vi "UpdateCurrent.vi"(8 "error in (no error)":errorcluster) -> (0 "error out":errorcluster)   [LabVIEW 2015]
uses:
  <vilib>/Rock Robotics/WPI/CAN/TalonSRX/WPI_CANTalonSRX_GlobalStatus.ctl
  Shooter Global.vi
panel:
  out "Set Pos":dbl(graph)
  out "Closed Loop Error":dbl(graph)
  out "Encoder Pos":dbl(graph)
  out "Current":dbl(graph)
  out "Talon SRX Status":T1
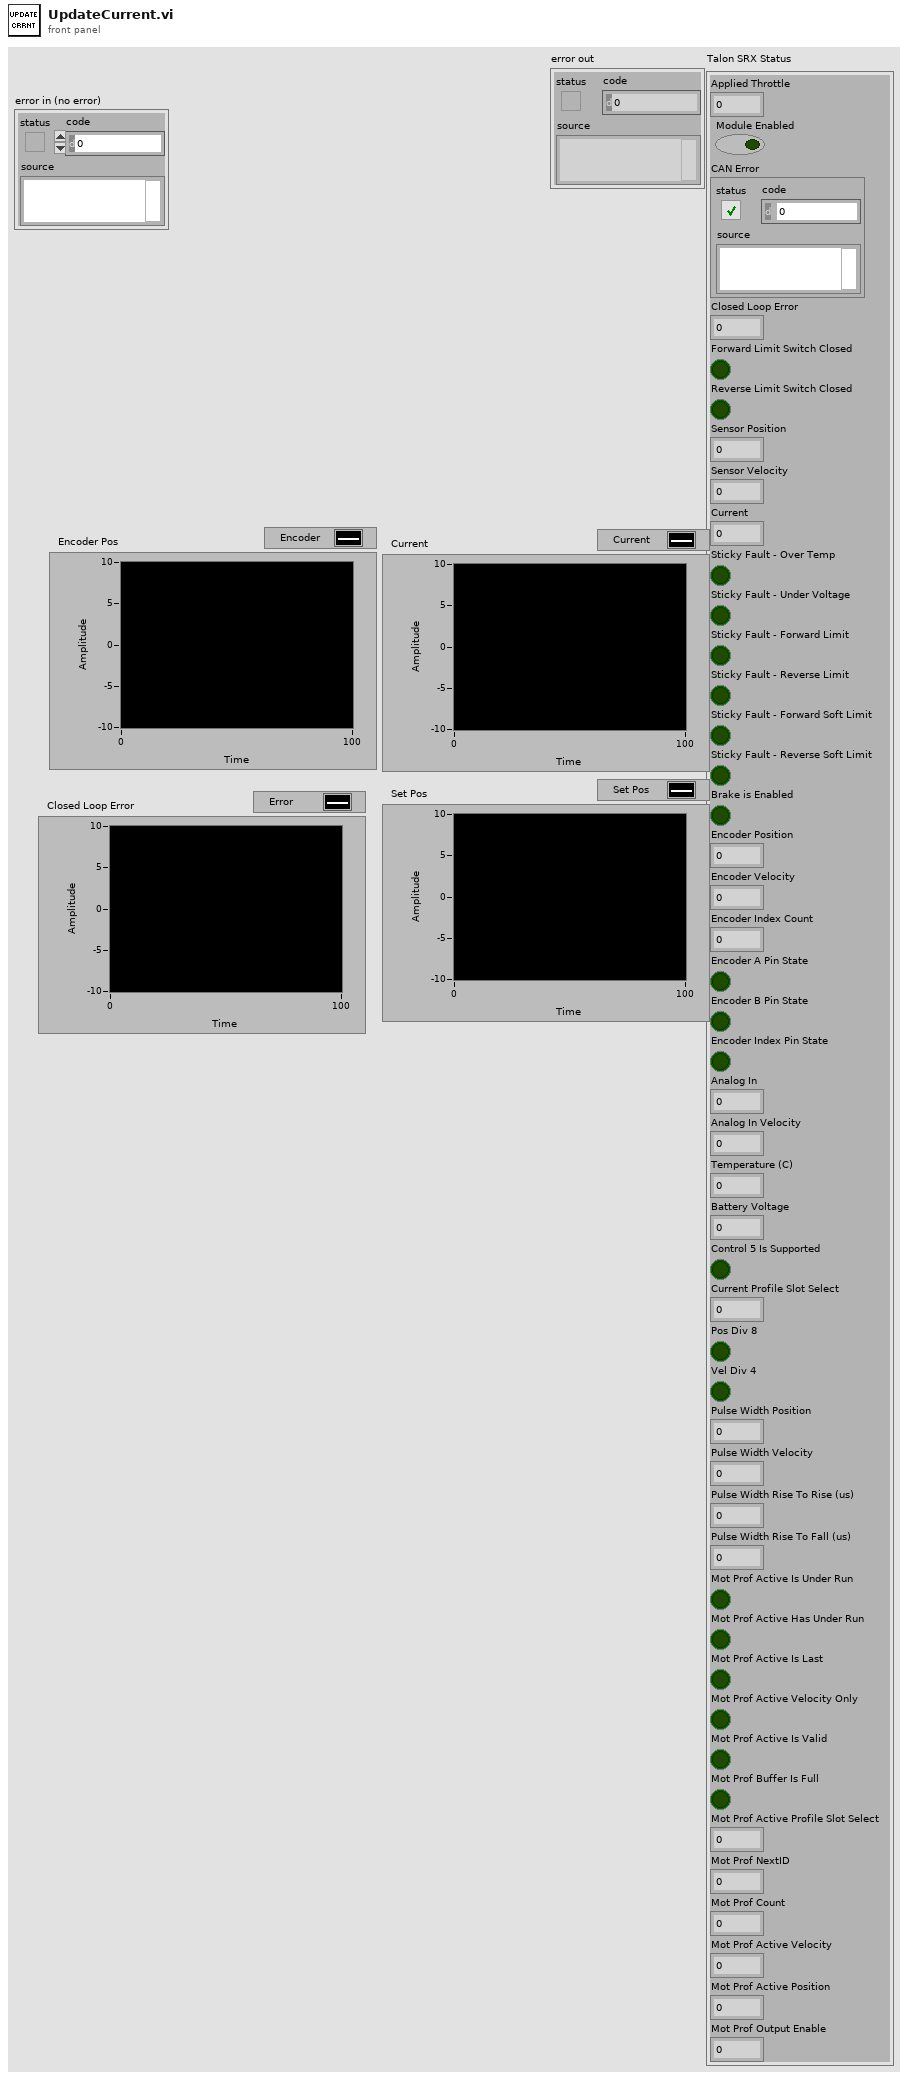
[diagram p1: front panel]
types:
  T1 = typedef "WPI_CANTalonSRX_GlobalStatus.ctl" = cluster{"Applied Throttle":dbl, "Module Enabled":bool, "CAN Error":errorcluster, "Closed Loop Error":dbl, "Forward Limit Switch Closed":bool, "Reverse Limit Switch Closed":bool, "Sensor Position":dbl, "Sensor Velocity":dbl, "Current":dbl, "Sticky Fault - Over Temp":bool, "Sticky Fault - Under Voltage":bool, "Sticky Fault - Forward Limit":bool, "Sticky Fault - Reverse Limit":bool, "Sticky Fault - Forward Soft Limit":bool, "Sticky Fault - Reverse Soft Limit":bool, "Brake is Enabled":bool, "Encoder Position":dbl, "Encoder Velocity":dbl, "Encoder Index Count":dbl, "Encoder A Pin State":bool, "Encoder B Pin State":bool, "Encoder Index Pin State":bool, "Analog In":dbl, "Analog In Velocity":dbl, "Temperature (C)":dbl, "Battery Voltage":dbl, "Control 5 Is Supported":bool, "Current Profile Slot Select":dbl, "Pos Div 8":bool, "Vel Div 4":bool, "Pulse Width Position":i32, "Pulse Width Velocity":i32, "Pulse Width Rise To Rise (us)":i32, "Pulse Width Rise To Fall (us)":i32, "Mot Prof Active Is Under Run":bool, "Mot Prof Active Has Under Run":bool, "Mot Prof Active Is Last":bool, "Mot Prof Active Velocity Only":bool, "Mot Prof Active Is Valid":bool, "Mot Prof Buffer Is Full":bool, "Mot Prof Active Profile Slot Select":i32, "Mot Prof NextID":i32, "Mot Prof Count":i32, "Mot Prof Active Velocity":dbl, "Mot Prof Active Position":dbl, "Mot Prof Output Enable":i32}
  T2 = typedef "Arm Settings Type Def.ctl" = cluster{"Min Arm Pos":dbl, "Max Arm Pos":dbl, "Drive Pos":dbl, "Arm Increments":dbl, "Obstacle Pos":dbl, "Max Current":dbl}
  T3 = typedef "Detailed Motor Type Def.ctl" = cluster{"MotorRef":T4, "Encoder Ticks Per Rev":dbl, "Set Position":dbl, "Wheel Radius":dbl}
  T4 = typedef "WPI_MotorControlDeviceRef.ctl" = cluster{"DeviceStatus":errorcluster, "Type":T5, "PWM":cluster{"PWM Channel":T6, "DeadBand":T7}, "CAN":cluster{"Device Number":u8, "Control Mode":T8, "Semaphore":T9, "Max Vout":dbl, "TalonSRX Control Mode":T10}, "Invert":bool}
  T5 = typedef "WPI_MotorControlType.ctl" = enum16{"PWM", "CAN", "CANTalonSRX"}
  T6 = typedef "FPGA_DIOPWMChannel.ctl" = enum8{"PWM 0", "PWM 1", "PWM 2", "PWM 3", "PWM 4", "PWM 5", "PWM 6", "PWM 7", "PWM 8", "PWM 9", "PWM MXP 0", "PWM MXP 1", "PWM MXP 2", "PWM MXP 3", "PWM MXP 4", "PWM MXP 5", "PWM MXP 6", "PWM MXP 7", "PWM MXP 8", "PWM MXP 9", "Invalid"}
  T7 = typedef "WPI_PWMDeadband.ctl" = cluster{"Name":string, "maxPositivePwm":i32, "minPositivePwm":i32, "centerPwm":i32, "maxNegativePwm":i32, "minNegativePwm":i32, "angularRange":u16}
  T8 = typedef "WPI_CANJaguar_ControlMode.ctl" = enum8{"Percent VBus", "Current", "Speed", "Position", "Voltage"}
  T9 = typedef "Semaphore RefNum" = refnum<k1>
  T10 = typedef "WPI_CANTalonSRX_APIControlMode.ctl" = enum8{"Percent VBus", "Speed", "Position", "Slave", "Unchanged / Invalid", "Voltage Compensation", "Current", "Motion Profile"}
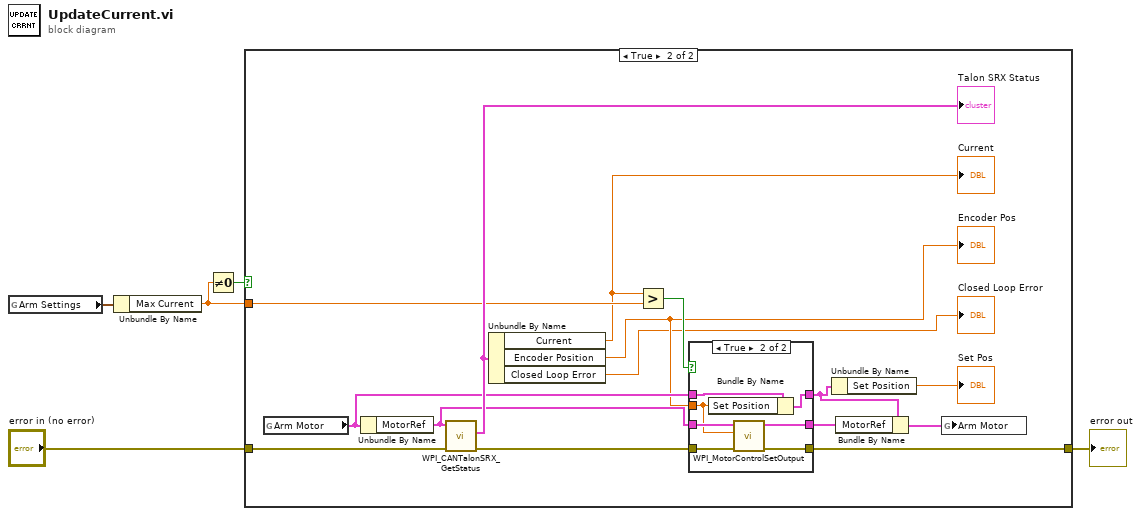
[diagram p0: block diagram]
diagram:
  n1 = global read "Shooter Global.vi" "Arm Settings"() -> (w5:T2)
  n2 = Unbundle By Name(w5) -> ("Max Current"=w3:dbl)
  n3 = Not Equal To 0?(x=w3) -> (x != 0?=w4:bool)
  n4 = case shown="True" w4 {
    tunnel: w3 -> [_ w15]
    tunnel: "error in (no error)" -> [w6 w13]
    tunnel: [w6 w12] -> w1
    frame False {
    }
    frame True {
      n5 = global read "Shooter Global.vi" "Arm Motor"() -> (w14:T3)
      n6 = Unbundle By Name(w14) -> ("MotorRef"=w19:T4)
      n7 = call <vilib>:"WPI_CANTalonSRX_GetStatus.vi"("error in (no error)"=w13, "CAN Talon SRX Ref"=w19) -> ("error out"=w18:errorcluster, "Talon SRX Status"=w21:T1)  [unwired: 7 in, 1 out]
      "Talon SRX Status" <- w21
      n8 = Unbundle By Name(w21) -> ("Current"=w10:dbl, "Encoder Position"=w9:dbl, "Closed Loop Error"=→"Closed Loop Error":dbl)
      "Current" <- w10
      "Encoder Pos" <- w9
      n9 = Greater?(x=w10, y=w15) -> (0:w20:bool)
      n10 = case shown="True" w20 {
        tunnel: w9 -> [_ w25]
        tunnel: w19 -> [w23 w31]
        tunnel: w18 -> [w24 w30]
        tunnel: [w24 w29] -> w12
        tunnel: [w23 w28] -> w17
        tunnel: w14 -> [w22 w27]
        tunnel: [w22 w26] -> w11
        frame False {
        }
        frame True {
          n11 = Bundle By Name(cluster=w27, "Set Position"=w25) -> (w26:T3)
          n12 = call <vilib>:"WPI_MotorControlSetOutput.vi"("error in (no error)"=w30, "Output"=w25, "MotorControlDevRef"=w31) -> ("error out"=w29:errorcluster, "MotorControlDevRef"=w28:T4)  [unwired: 6 in, 1 out]
        }
      }
      n13 = Unbundle By Name(w11) -> ("Set Position"=→"Set Pos":dbl)
      n14 = Bundle By Name(cluster=w11, "MotorRef"=w17) -> (w16:T3)
      n15 = global write "Shooter Global.vi" "Arm Motor"(w16) -> ()
    }
  }
  "error out" <- w1
